vi "ZY_Relay_OFF.vi"(7 "COM":refnum<visa-resource-name>, 8 "error in (no error)":errorcluster, 11 "Limit in":string) -> (0 "error out":errorcluster, 2 "Result":bool, 3 "String":string)   [LabVIEW 2013]
panel:
  # "1@~1~2~3~4\nAdd@~ch~ch~ch"
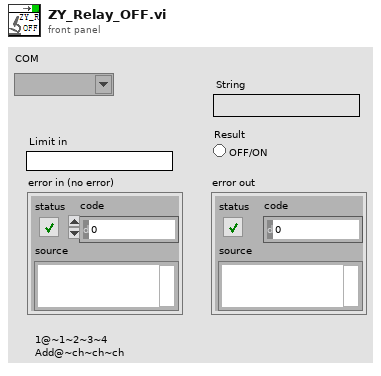
[diagram p1: front panel]
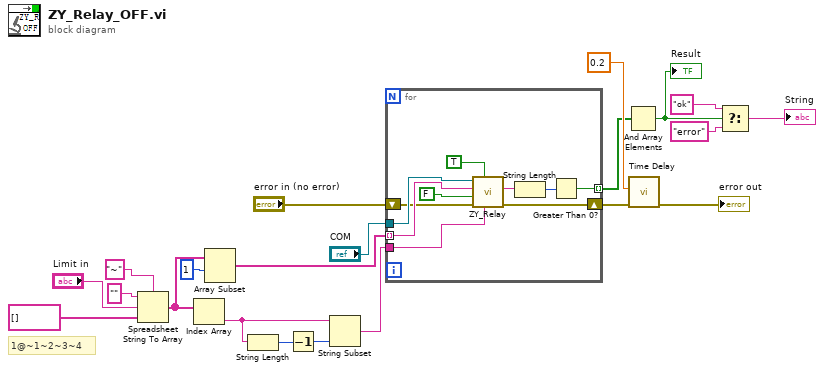
[diagram p0: block diagram]
diagram:
  # "1@~1~2~3~4"
  n1 = Spreadsheet String To Array(delimiter (Tab)="~", format string="", spreadsheet string="Limit in", array type (2D Dbl)=string[] []) -> (array=w3:string[])
  n2 = Index Array(array=w3) -> (element=w7:string)  [unwired: 1 in]
  n3 = Array Subset(array=w3, index=1) -> (w2:string[])  [unwired: 1 in]
  n4 = String Length(string=w7) -> (length=w6:i32)
  n5 = Decrement(x=w6) -> (x-1=w5:i32)
  n6 = String Subset(string=w7, length (rest)=w5) -> (substring=w1:string)  [unwired: 1 in]
  n7 = for {
    tunnel: w2 -> [w30] mode=indexing
    shift-right: [w27] -> w14
    shift-left: "error in (no error)" -> [w28]
    tunnel: "COM" -> [w31]
    tunnel: [w23] -> w9 mode=indexing
    tunnel: w1 -> [w22]
    n8 = call "ZY_Relay.vi"("Addr"=w22, "Read?"=TRUE, "error in (no error)"=w28, "ON?"=FALSE, "Channel"=w30, "VISA resource name"=w31) -> ("error out"=w27:errorcluster, "read buffer"=w25:string)  [unwired: 4 in]
    n9 = String Length(string=w25) -> (length=w24:i32)
    n10 = Greater Than 0?(x=w24) -> (x > 0?=w23:bool)
  }
  n11 = And Array Elements(Boolean array=w9) -> (logical AND=w8:bool)
  "Result" <- w8
  n12 = call "Time Delay"("error in (no error)"=w14, "Delay Time (s)"=0.2) -> ("error out"=→"error out":errorcluster)  [unwired: 9 in]
  n13 = Select(t="ok", s=w8, f="error") -> (s? t:f=→"String":string)
